vi "ELVIS III v1.1 Stop AI Continuous.vi"(8 "error in (no error)":errorcluster, 10 "Bank Count":u8[](array[numeric]), 11 "AI (Continuous) Ref In":T1) -> (0 "error out":errorcluster, 3 "AI (Continuous) Ref Out":T1)   [LabVIEW 2021]
uses:
  <vilib>/myRIO/Common/Instrument Driver Framework/Utilities/typedefs/myRIO v1.0 Reference.ctl
  <vilib>/myRIO/Common/Instrument Driver Framework/Utilities/typedefs/Generic FPGA Reference.ctl
  <vilib>/myRIO/Common/Instrument Driver Framework/ELVIS III v1.0/AI Block/typedefs/ELVIS III AI Block Channels FPGA Reference.ctl
  <vilib>/Utility/error.llb/Error Cluster From Error Code.vi
  <vilib>/rvi/errors/niLvFpgaAdjustHostInterfaceError.vi
  <vilib>/rvi/interface/nirviReadWriteControl/nirviReadWriteControl.xnode
  NiFpgaLv.dll
  <vilib>/rvi/interface/Simulation/niFpgaSimulationCallBeginRW.vi
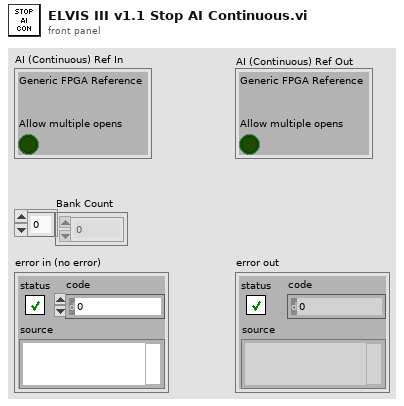
[diagram p1: front panel]
types:
  T1 = typedef "myRIO v1.0 Reference.ctl" = cluster{"Generic FPGA Reference":T2, "Allow multiple opens":bool}
  T2 = typedef "Generic FPGA Reference.ctl" = refnum<k20>
  T3 = typedef "ELVIS III AI Block Channels FPGA Reference.ctl" = refnum<k20>
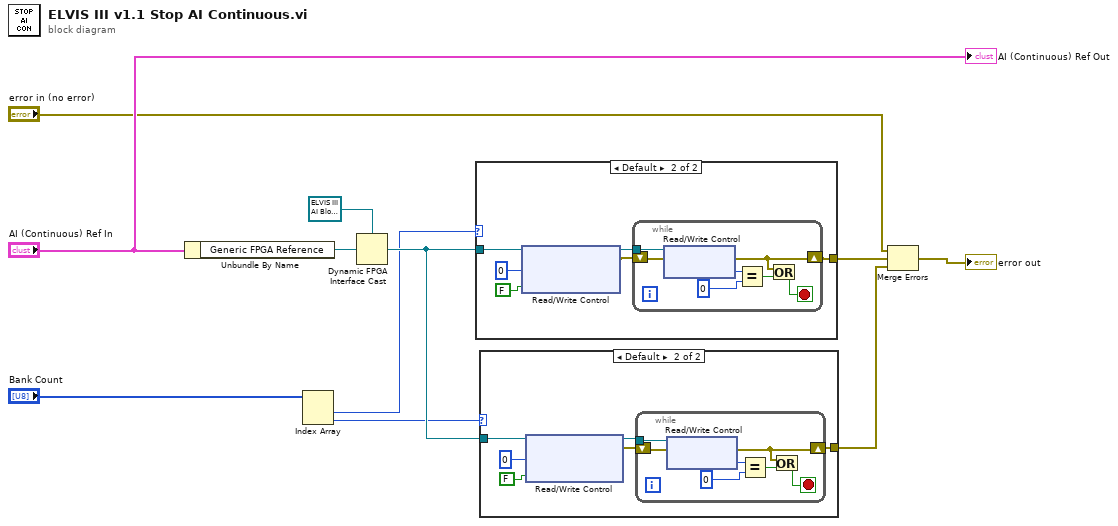
[diagram p0: block diagram]
diagram:
  n1 = Unbundle By Name("AI (Continuous) Ref In") -> ("Generic FPGA Reference"=w7:T2)
  n2 = Index Array(array="Bank Count") -> (element #1=w3:u8, element #2=w2:u8)  [unwired: 2 in]
  n3 = Dynamic FPGA Interface Cast(Session In=T3 refnum ("AI Block Channels FPGA Reference"), Type=w7) -> (Session Out=w6:T3)
  n4 = case shown="Default" w3 {
    tunnel: w6 -> [_ w15]
    tunnel: [_ w13] -> w5
    frame 0 {
    }
    frame Default {
      n5 = xnode "Read/Write Control"("FPGA VI Reference In"=w15, "AI.A.CNT"=u8 0 ("AI.B.CNT"), "AI.A.DMA_ENA"=FALSE ("AI.B.DMA_ENA")) -> ("FPGA VI Reference Out"=w12:T3, "error out"=w14:errorcluster)  [unwired: 1 in]
      n6 = while {
        tunnel: w12 -> [w24]
        shift-right: [w18] -> w13
        shift-left: w14 -> [w23]
        stop <- w19 stop-if-true
        n7 = xnode "Read/Write Control"("FPGA VI Reference In"=w24, "error in"=w23) -> ("error out"=w18:errorcluster, "AI.A.STAT"=w22:u8)  [unwired: 1 out]
        n8 = Equal?(x=w22, y=u8 0) -> (x = y?=w20:bool)
        n9 = Or(x=w18, y=w20) -> (x .or. y?=w19:bool)
      }
    }
  }
  n10 = case shown="Default" w2 {
    tunnel: w6 -> [_ w28]
    tunnel: [_ w25] -> w4
    frame 0 {
    }
    frame Default {
      n11 = xnode "Read/Write Control"("FPGA VI Reference In"=w28, "AI.B.CNT"=u8 0, "AI.B.DMA_ENA"=FALSE) -> ("FPGA VI Reference Out"=w27:T3, "error out"=w26:errorcluster)  [unwired: 1 in]
      n12 = while {
        tunnel: w27 -> [w37]
        shift-right: [w31] -> w25
        shift-left: w26 -> [w36]
        stop <- w32 stop-if-true
        n13 = xnode "Read/Write Control"("FPGA VI Reference In"=w37, "error in"=w36) -> ("error out"=w31:errorcluster, "AI.B.STAT"=w35:u8)  [unwired: 1 out]
        n14 = Equal?(x=w35, y=u8 0) -> (x = y?=w33:bool)
        n15 = Or(x=w31, y=w33) -> (x .or. y?=w32:bool)
      }
    }
  }
  n16 = Merge Errors("error in (no error)", w5, w4) -> (→"error out":errorcluster)
  "AI (Continuous) Ref Out" <- "AI (Continuous) Ref In"
